vi "Read Connection Information.vi"(8 "error in (no error)":errorcluster, 11 "TwinCAT ADS in":refnum<class "TwinCAT ADS.lvclass">) -> (0 "error out":errorcluster, 1 "Connection Information":T1 {"ConnectionState" items=["None, Unknown", "Disconnected", "Connected", "Lost"]; "Router State" items=["Stop"=0, "Start"=1, "Removed"=2, "Unknown"=-1]; "Protocol" items=["None", "Router", "TcpIp", "All"]}, 3 "TwinCAT ADS out":refnum<class "TwinCAT ADS.lvclass">)   [LabVIEW 2018, in "TwinCAT ADS.lvclass"]
uses:
  TwinCAT ADS.lvclass
  Controls/Connection Information.ctl
  TwinCAT.Ads
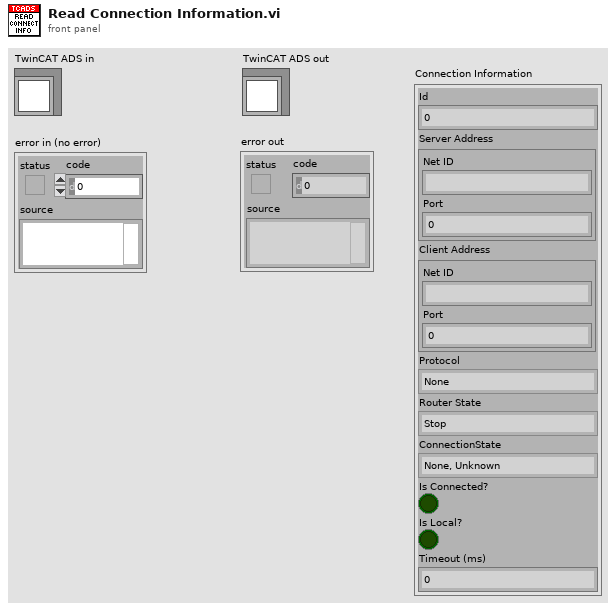
[diagram p1: front panel]
types:
  T1 = typedef "TwinCAT ADS.lvclass/Connection Information.ctl" = cluster{"Id":i32, "Server Address":cluster{"Net ID":string, "Port":i32}, "Client Address":cluster{"Net ID":string, "Port":i32}, "Protocol":i32, "Router State":i32, "ConnectionState":i32, "Is Connected?":bool, "Is Local?":bool, "Timeout (ms)":i32}
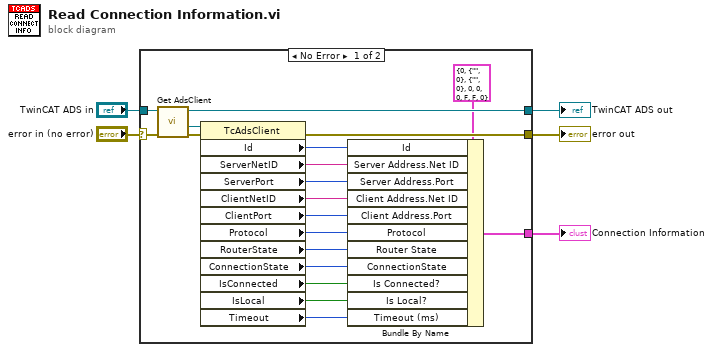
[diagram p0: block diagram]
diagram:
  n1 = case shown="No Error" "error in (no error)" {
    selector: "error in (no error)" -> [w11 w26]
    tunnel: [w24 w26] -> w4
    tunnel: [w7 w25] -> w2
    tunnel: "TwinCAT ADS in" -> [w8 w25]
    tunnel: [w12 _] -> w1
    frame No Error {
      n2 = call-dynamic "Get AdsClient.vi"("error in (no error)"=w11, "TwinCAT ADS in"=w8) -> ("error out"=w10:errorcluster, ".NET TcAdsClient refnum"=w9:refnum<k24>, "TwinCAT ADS out"=w7:refnum<class "TwinCAT ADS.lvclass">)  [unwired: 7 in]
      n3 = property class="TcAdsClient"(reference=w9, error in=w10) -> (error out=w24:errorcluster, "Id"=w23:i32, "ServerNetID"=w22:string, "ServerPort"=w21:i32, "ClientNetID"=w20:string, "ClientPort"=w19:i32, "Protocol"=w18:i32, "RouterState"=w17:i32, "ConnectionState"=w13:i32, "IsConnected"=w14:bool, "IsLocal"=w15:bool, "Timeout"=w16:i32)  [unwired: 1 out]
      n4 = Bundle By Name(cluster=T1 {"Id"=0, "Server Address"={"Net ID"="", "Port"=0}, "Client Address"={"Net ID"="", "Port"=0}, "Protocol"=0, "Router State"=0, "ConnectionState"=0, "Is Connected?"=FALSE, "Is Local?"=FALSE, "Timeout (ms)"=0} ("Connectio Information"), "Id"=w23, "Server Address.Net ID"=w22, "Server Address.Port"=w21, "Client Address.Net ID"=w20, "Client Address.Port"=w19, "Protocol"=w18, "Router State"=w17, "ConnectionState"=w13, "Is Connected?"=w14, "Is Local?"=w15, "Timeout (ms)"=w16) -> (w12:T1)
    }
    frame Error {
    }
  }
  "error out" <- w4
  "TwinCAT ADS out" <- w2
  "Connection Information" <- w1
